vi "WVDIAL_GlobalVariables.vi"() -> ()   [LabVIEW 2024]
uses:
  TypeDefinitions.llb/TypeDef_MainControlSystem.ctl
  TypeDefinitions.llb/TypeDef_MainSpecialConfiguration.ctl
panel:
  in  "Configuration":T1
  in  "ChildTimeout (sec)":dbl=5.0
  out "ChildAbort":bool
  in  "VI Timeout (min)":dbl=5.0
  out "RunAsChild":bool
  out "GlobalStop":bool
  in  "PermissionLevel":i32
  out "Children Details":T3(array[cluster])
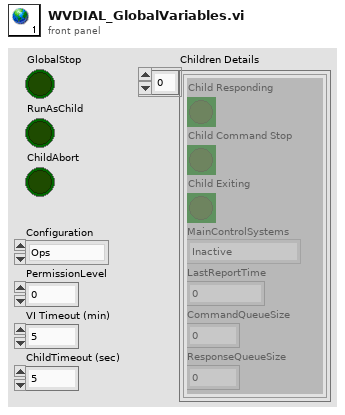
[diagram p1: front panel]
types:
  T1 = typedef "TypeDef_MainSpecialConfiguration.ctl" = enum16{"Ops", "ReceiverScan", "PulsedScan", "HyperFineScan"}
  T2 = typedef "TypeDef_MainControlSystem.ctl" = enum16{"Inactive", "MCS", "MCSControls", "LaserControl", "LaserLocking", "WeatherStation", "DataDisplay", "DataNetCDF", "Template", "WavelengthLocking", "Wavemeter", "Switches", "Thermocouple", "UPS", "PowerSwitches", "Thor8000", "ReceiverScan", "Clock", "HumiditySensor", "SetupReceiverScan", "ConfigureQC", "ConfigureThor8000", "Container", "CurrentSensor", "TCSPC", "Aerodiode", "Balanced Detector", "HVAC"}
  T3 = cluster{"Child Command Stop":bool, "Child Responding":bool, "MainControlSystems":T2, "LastReportTime":dbl, "Child Exiting":bool, "CommandQueueSize":dbl, "ResponseQueueSize":dbl}[]
diagram:
